vi "TestMeasurementTcpDataProcessing.vi"(10 "Address":string, 11 "Read Data":T3(array[cluster])) -> (2 "Data":T2, 3 "Read Data Out":T3(array[cluster]))   [LabVIEW 2021]
uses:
  HallMeasurementStatus.ctl
  TestFgvCMD.ctl
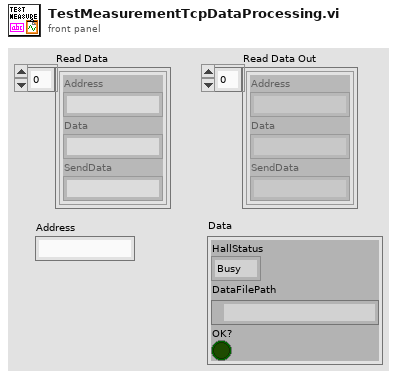
[diagram p1: front panel]
types:
  T1 = typedef "HallMeasurementStatus.ctl" = enum16{"Busy", "Ready", "Done", "Error"}
  T2 = cluster{"HallStatus":T1, "DataFilePath":path, "OK?":bool}
  T3 = cluster{"Address":string, "Data":string, "SendData":string}[]
  T4 = typedef "TestFgvCMD.ctl" = enum16{"Get", "Set", "SetOK?", "SetStatus", "SetDataPath"}
  T5 = typedef "TestMeasurementStatus.ctl" = enum16{"Busy", "Ready", "Done", "Error"}
  T6 = cluster{"Status":T5, "DataFilePath":path, "OK?":bool}
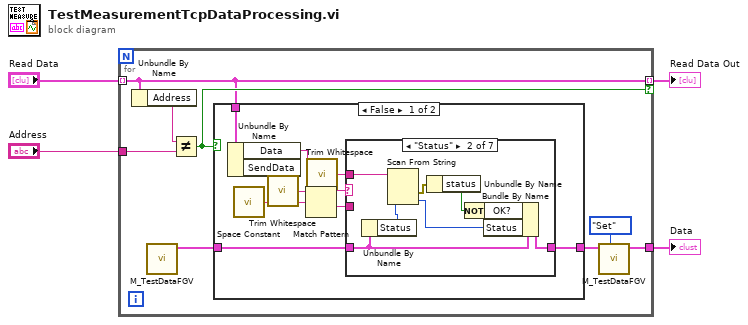
[diagram p0: block diagram]
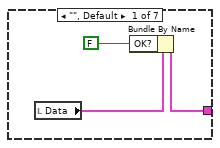
[diagram p2: hidden frame]
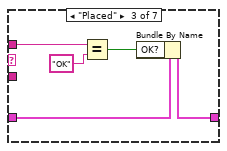
[diagram p3: hidden frame]
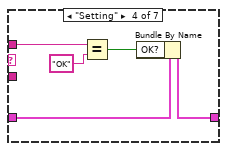
[diagram p4: hidden frame]
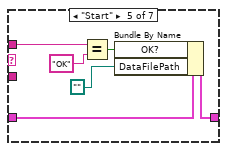
[diagram p5: hidden frame]
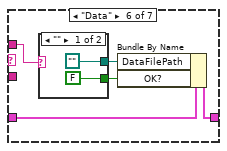
[diagram p6: hidden frame]
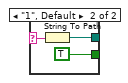
[diagram p7: hidden frame]
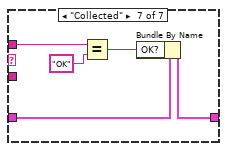
[diagram p8: hidden frame]
diagram:
  n1 = for {
    tunnel: "Read Data" -> [w9] mode=indexing
    tunnel: "Address" -> [w12]
    tunnel: [w9] -> w4 mode=indexing if=w10
    tunnel: [w5] -> w1
    n2 = Unbundle By Name(w9) -> ("Address"=w11:string)
    n3 = call "M_TestDataFGV.vi"() -> ("TestData Out"=w7:T6)  [unwired: 11 in]
    n4 = Not Equal?(x=w11, y=w12) -> (x != y?=w10:bool)
    n5 = case shown="False" w10 {
      tunnel: w9 -> [w22 _]
      tunnel: [w14 w65] -> w8
      tunnel: w7 -> [w13 w65]
      frame False {
        n6 = Unbundle By Name(w22) -> ("Data"=w16:string, "SendData"=w21:string)
        n7 = call <vilib>:"Space Constant.vi"() -> ("String"=w20:string)
        n8 = call <vilib>:"Trim Whitespace.vi"("string"=w21) -> ("trimmed string"=w19:string)  [unwired: 1 in]
        n9 = Match Pattern(string=w19, regular expression=w20) -> (before substring=w18:string, after substring=w17:string)  [unwired: 1 in, 2 out]
        n10 = call <vilib>:"Trim Whitespace.vi"("string"=w16) -> ("trimmed string"=w15:string)  [unwired: 1 in]
        n11 = case shown="\"Status\"" w18 {
          tunnel: w17 -> [_ _ _ _ _ _ _]
          tunnel: w15 -> [_ w32 w37 w42 w48 w52 w63]
          tunnel: [w25 w29 w35 w40 w46 w53 w60] -> w14
          tunnel: w13 -> [_ w30 w36 w41 w47 w54 w62]
          frame "", Default {
            n12 = local read "Data"() -> (w23:T2)
            n13 = Bundle By Name(cluster=w23, "OK?"=FALSE) -> (w25:T2)
          }
          frame "Status" {
            n14 = Unbundle By Name(w30) -> ("Status"=w31:T5)
            n15 = Scan From String(input string=w32, default 1=w31) -> (error out=w33:errorcluster, output 1=w28:T5)  [unwired: 3 in, 2 out]
            n16 = Unbundle By Name(w33) -> ("status"=w27:bool)
            n17 = Not(x=w27) -> (.not. x?=w26:bool)
            n18 = Bundle By Name(cluster=w30, "OK?"=w26, "Status"=w28) -> (w29:T6)
          }
          frame "Placed" {
            n19 = Equal?(x=w37, y="OK" ("Send Data")) -> (x = y?=w34:bool)
            n20 = Bundle By Name(cluster=w36, "OK?"=w34) -> (w35:T6)
          }
          frame "Setting" {
            n21 = Equal?(x=w42, y="OK" ("Send Data")) -> (x = y?=w39:bool)
            n22 = Bundle By Name(cluster=w41, "OK?"=w39) -> (w40:T6)
          }
          frame "Start" {
            n23 = Equal?(x=w48, y="OK" ("Send Data")) -> (x = y?=w45:bool)
            n24 = Bundle By Name(cluster=w47, "OK?"=w45, "DataFilePath"=path "") -> (w46:T6)
          }
          frame "Data" {
            n25 = case shown="\"\"" w52 {
              selector: w52 -> [_ w58]
              tunnel: [FALSE TRUE] -> w50
              tunnel: [path "" w57] -> w51
              frame "" {
              }
              frame "1", Default {
                n26 = String To Path(string=w58) -> (path=w57:path)
              }
            }
            n27 = Bundle By Name(cluster=w54, "DataFilePath"=w51, "OK?"=w50) -> (w53:T6)
          }
          frame "Collected" {
            n28 = Equal?(x=w63, y="OK" ("Send Data")) -> (x = y?=w61:bool)
            n29 = Bundle By Name(cluster=w62, "OK?"=w61) -> (w60:T6)
          }
        }
      }
      frame True {
      }
    }
    n30 = call "M_TestDataFGV.vi"("TestFgvCMD"=TestFgvCMD."Set" ("EllipsoFgvCMD"), "TestData In"=w8) -> ("TestData Out"=w5:T6)  [unwired: 9 in]
  }
  "Read Data Out" <- w4
  "Data" <- w1
